vi "Signal Generator.vi"(1 "Signal Properties":T1, 2 "Points":cluster{"X":dbl, "Y":dbl}[](array[cluster])) -> (0 "Signal":dbl[](array[numeric]))   [LabVIEW 2013]
uses:
  <vilib>/measure/NI_MABase.lvlib
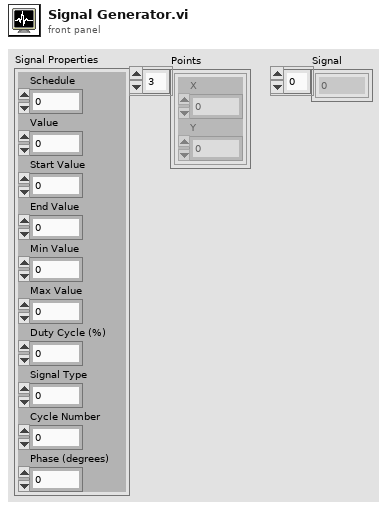
[diagram p1: front panel]
types:
  T1 = cluster{"Schedule":u16, "Value":dbl, "Start Value":dbl, "End Value":dbl, "Min Value":dbl, "Max Value":dbl, "Duty Cycle (%)":dbl, "Signal Type":u16, "Cycle Number":dbl, "Phase (degrees)":dbl}
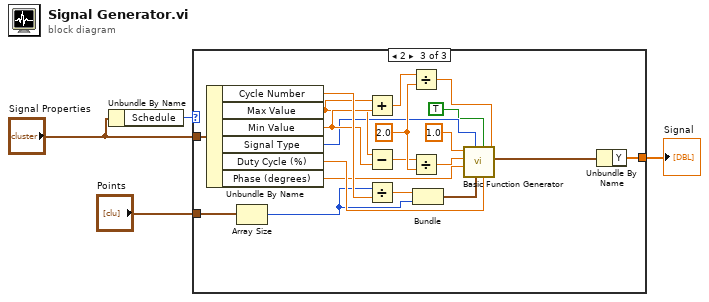
[diagram p0: block diagram]
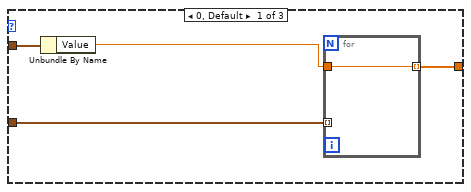
[diagram p2: hidden frame]
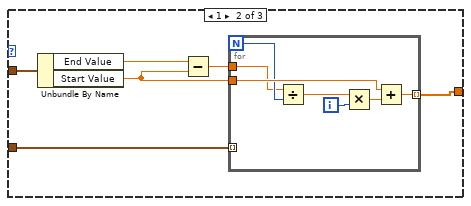
[diagram p3: hidden frame]
diagram:
  n1 = Unbundle By Name("Signal Properties") -> ("Schedule"=w3:u16)
  n2 = case shown="2" w3 {
    tunnel: "Signal Properties" -> [w8 w14 w42]
    tunnel: "Points" -> [w7 w15 w26]
    tunnel: [w5 w10 w41] -> w4
    frame 0, Default {
      n3 = Unbundle By Name(w8) -> ("Value"=w6:dbl)
      n4 = for {
        tunnel: w7 -> [_] mode=indexing
        tunnel: w6 -> [w9]
        tunnel: [w9] -> w5 mode=indexing
      }
    }
    frame 1 {
      n5 = Unbundle By Name(w14) -> ("End Value"=w13:dbl, "Start Value"=w11:dbl)
      n6 = Subtract(x=w13, y=w11) -> (x-y=w12:dbl)
      n7 = for {
        N -> [w17]
        tunnel: w15 -> [_] mode=indexing
        tunnel: w12 -> [w16]
        tunnel: w11 -> [w20]
        tunnel: [w19] -> w10 mode=indexing
        i -> [w22]
        n8 = Divide(x=w16, y=w17) -> (x/y=w18:dbl)
        n9 = Multiply(x=w18, y=w22) -> (x*y=w21:dbl)
        n10 = Add(x=w20, y=w21) -> (x+y=w19:dbl)
      }
    }
    frame 2 {
      w36 = 2.0 ("y")
      n11 = Unbundle By Name(w42) -> ("Cycle Number"=w39:dbl, "Max Value"=w33:dbl, "Min Value"=w34:dbl, "Signal Type"=w32:u16, "Duty Cycle (%)"=w38:dbl, "Phase (degrees)"=w27:dbl)
      n12 = Array Size(array=w26) -> (size(s)=w25:i32)
      n13 = Add(x=w33, y=w34) -> (x+y=w30:dbl)
      n14 = Subtract(x=w33, y=w34) -> (x-y=w35:dbl)
      n15 = Divide(x=w25, y=w39) -> (x/y=w40:dbl)
      n16 = Divide(x=w30, y=w36) -> (x/y=w31:dbl)
      n17 = Divide(x=w35, y=w36) -> (x/y=w37:dbl)
      n18 = Bundle(w40, w25) -> (w24:cluster{dbl, i32})  [unwired: 1 in]
      n19 = call <vilib>:"Basic Function Generator.vi"("offset"=w31, "square wave duty cycle (%)"=w38, "reset signal"=TRUE, "sampling info"=w24, "signal type"=w32, "phase"=w27, "amplitude"=w37, "frequency"=1.0) -> ("signal out"=w28:waveform(dbl))  [unwired: 1 in, 2 out]
      n20 = Unbundle By Name(w28) -> ("Y"=w41:dbl[])
    }
  }
  "Signal" <- w4
